vi "Dispose.vi"(8 "error in (no error)":errorcluster, 11 "Actor in":refnum<class "Actor.lvclass">) -> (0 "error out":errorcluster, 3 "Actor out":refnum<class "Actor.lvclass">)   [LabVIEW 2020, in "CameraTestingUI.lvlib" / "CameraTestingUI.lvclass"]
uses:
  CameraTestingUI.lvclass
  <vilib>/ActorFramework/Actor/Actor.lvclass
  C:/Program Files (x86)/National Instruments/LabVIEW 2020/vi.lib/ActorFramework/Actor/Actor.lvclass
  CameraTestingUI.lvclass/CameraTestingUI.ctl
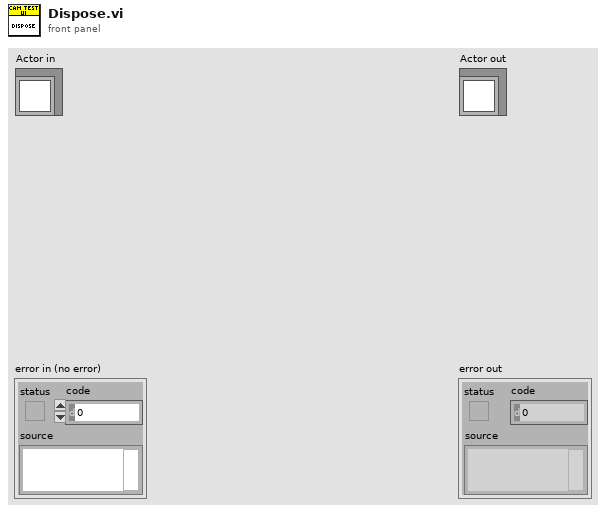
[diagram p1: front panel]
types:
  T1 = typedef "CameraTestingUI.lvlib/CameraTestingUI.lvclass/UpdCamTestEvntRegRef.ctl" = refnum<user-event>
  T2 = typedef "CameraTestingUI.lvlib/CameraTestingUI.lvclass/QuitActorEvn.ctl" = refnum<user-event>
  T3 = typedef "CameraTestingUI.lvlib/CameraTestingUI.lvclass/HelperLoopEvntRegRef.ctl" = refnum<event-registration>
  T4 = typedef "CameraTestingUI.lvlib/CameraTestingUI.lvclass/VideoLoopEnvRgstRef.ctl" = refnum<event-registration>
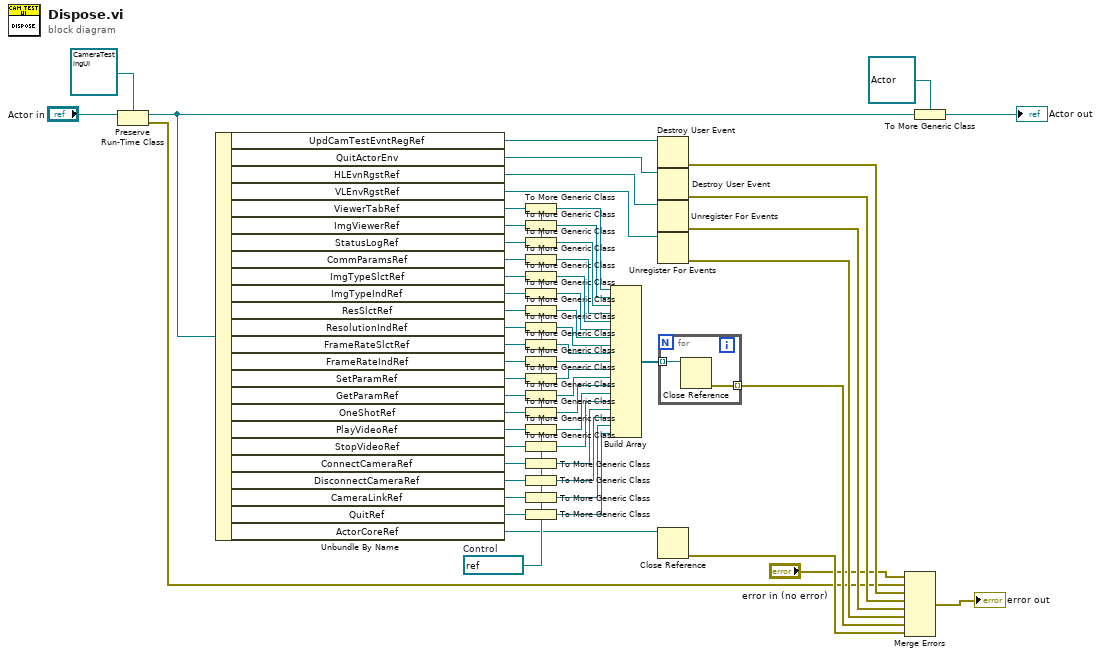
[diagram p0: block diagram]
diagram:
  w30 = refnum<vi> refnum  # Control
  n1 = Preserve Run-Time Class(object in="Actor in", 2:refnum<class "CameraTestingUI.lvclass"> refnum ("CameraTestingUI.lvlib:CameraTestingUI.lvclass")) -> (object out=w53:refnum<class "CameraTestingUI.lvclass">, error out=w2:errorcluster)  [unwired: 1 in]
  n2 = Unbundle By Name(w53) -> ("UpdCamTestEvntRegRef"=w59:T1, "QuitActorEnv"=w58:T2, "HLEvnRgstRef"=w57:T3, "VLEnvRgstRef"=w56:T4, "ViewerTabRef"=w49:refnum<vi>, "ImgViewerRef"=w48:refnum<vi>, "StatusLogRef"=w47:refnum<vi>, "CommParamsRef"=w46:refnum<vi>, "ImgTypeSlctRef"=w45:refnum<vi>, "ImgTypeIndRef"=w44:refnum<vi>, "ResSlctRef"=w43:refnum<vi>, "ResolutionIndRef"=w42:refnum<vi>, "FrameRateSlctRef"=w41:refnum<vi>, "FrameRateIndRef"=w40:refnum<vi>, "SetParamRef"=w39:refnum<vi>, "GetParamRef"=w38:refnum<vi>, "OneShotRef"=w37:refnum<vi>, "PlayVideoRef"=w36:refnum<vi>, "StopVideoRef"=w35:refnum<vi>, "ConnectCameraRef"=w34:refnum<vi>, "DisconnectCameraRef"=w33:refnum<vi>, "CameraLinkRef"=w32:refnum<vi>, "QuitRef"=w31:refnum<vi>, "ActorCoreRef"=w9:refnum<vi>)
  n3 = To More Generic Class(target class=w30, reference=w49) -> (generic class reference=w29:refnum<vi>)
  n4 = To More Generic Class(target class=w30, reference=w48) -> (generic class reference=w28:refnum<vi>)
  n5 = To More Generic Class(target class=w30, reference=w47) -> (generic class reference=w27:refnum<vi>)
  n6 = To More Generic Class(target class=w30, reference=w46) -> (generic class reference=w26:refnum<vi>)
  n7 = To More Generic Class(target class=w30, reference=w45) -> (generic class reference=w25:refnum<vi>)
  n8 = To More Generic Class(target class=w30, reference=w44) -> (generic class reference=w24:refnum<vi>)
  n9 = To More Generic Class(target class=w30, reference=w43) -> (generic class reference=w23:refnum<vi>)
  n10 = To More Generic Class(target class=w30, reference=w42) -> (generic class reference=w22:refnum<vi>)
  n11 = To More Generic Class(target class=w30, reference=w41) -> (generic class reference=w21:refnum<vi>)
  n12 = To More Generic Class(target class=w30, reference=w40) -> (generic class reference=w20:refnum<vi>)
  n13 = To More Generic Class(target class=w30, reference=w39) -> (generic class reference=w19:refnum<vi>)
  n14 = To More Generic Class(target class=w30, reference=w38) -> (generic class reference=w18:refnum<vi>)
  n15 = To More Generic Class(target class=w30, reference=w37) -> (generic class reference=w17:refnum<vi>)
  n16 = To More Generic Class(target class=w30, reference=w36) -> (generic class reference=w16:refnum<vi>)
  n17 = To More Generic Class(target class=w30, reference=w35) -> (generic class reference=w15:refnum<vi>)
  n18 = To More Generic Class(target class=w30, reference=w34) -> (generic class reference=w14:refnum<vi>)
  n19 = To More Generic Class(target class=w30, reference=w33) -> (generic class reference=w13:refnum<vi>)
  n20 = To More Generic Class(target class=w30, reference=w32) -> (generic class reference=w12:refnum<vi>)
  n21 = To More Generic Class(target class=w30, reference=w31) -> (generic class reference=w11:refnum<vi>)
  n22 = Build Array(w29, w28, w27, w26, w25, w24, w23, w22, w21, w20, w19, w18, w17, w16, w15, w14, w13, w12, w11) -> (w10:refnum<vi>[])
  n23 = Destroy User Event(user event=w59) -> (error out=w3:errorcluster)  [unwired: 1 in]
  n24 = Destroy User Event(user event=w58) -> (error out=w4:errorcluster)  [unwired: 1 in]
  n25 = Unregister For Events(event registration refnum=w57) -> (error out=w5:errorcluster)  [unwired: 1 in]
  n26 = Unregister For Events(event registration refnum=w56) -> (error out=w6:errorcluster)  [unwired: 1 in]
  n27 = Close Reference(reference=w9) -> (error out=w8:errorcluster)  [unwired: 1 in]
  n28 = for {
    tunnel: w10 -> [w61] mode=indexing
    tunnel: [w60] -> w7 mode=indexing
    n29 = Close Reference(reference=w61) -> (error out=w60:errorcluster)  [unwired: 1 in]
  }
  n30 = Merge Errors("error in (no error)", w2, w3, w4, w5, w6, w7, w8) -> (→"error out":errorcluster)
  n31 = To More Generic Class(target class=refnum<class "Actor.lvclass"> refnum ("Actor in"), reference=w53) -> (generic class reference=→"Actor out":refnum<class "Actor.lvclass">)
